vi "Test.vi"() -> ()   [LabVIEW 2015, in "PolyVIEW.lvclass"]
uses:
  PolyVIEW.lvclass
  actors/world/typedefs/markValue.ctl
  actors/world/world.lvlib
  actors/world/typedefs/markVolume.ctl
  actors/world/typedefs/markValue_cluster.ctl
  actors/world/typedefs/amountOfFood.ctl
  actors/world/typedefs/anthillType_enum.ctl
  actors/world/typedefs/worldCell_cluster.ctl
panel:
  out "Waveform Graph 3":dbl[](graph)
  out "Waveform Graph":dbl[](graph)
  out "Waveform Graph 2":dbl[][](graph)
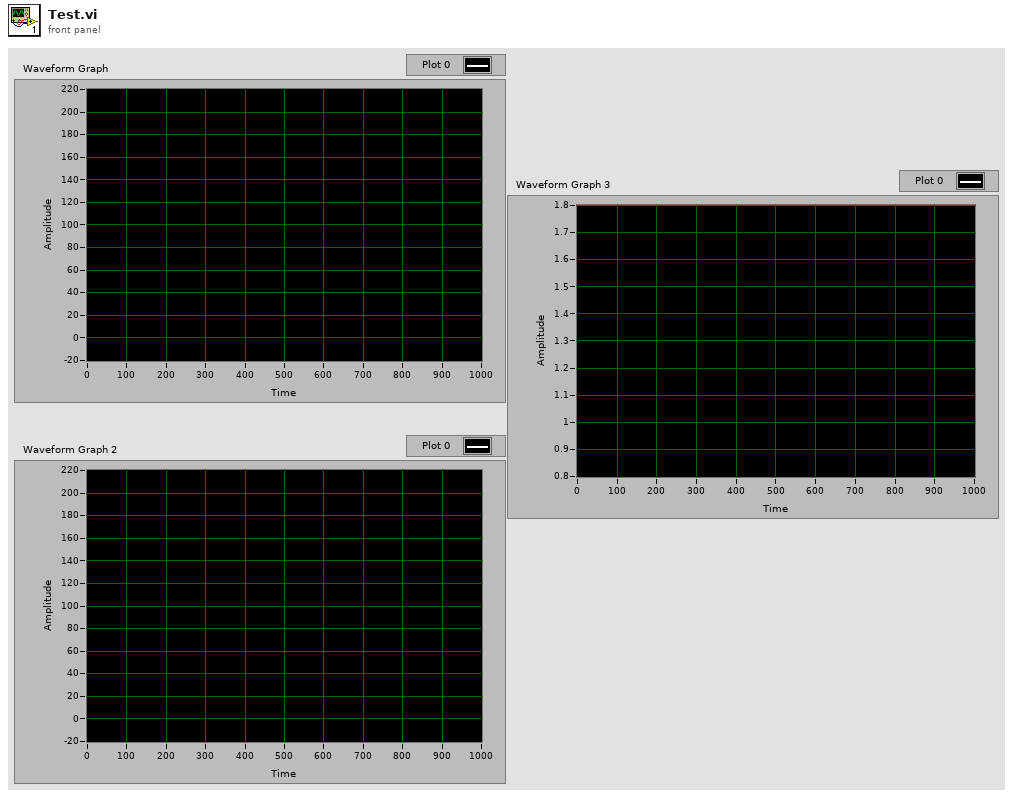
[diagram p1: front panel]
types:
  T1 = typedef "world.lvlib/worldCell_cluster.ctl" = cluster{"marksArray":T2[], "foodAmount":T5, "anthillType":T6, "absoluteHeight":u8}
  T2 = typedef "world.lvlib/markValue_cluster.ctl" = cluster{"value":T3, "volume":T4}
  T3 = typedef "world.lvlib/markValue.ctl" = u8
  T4 = typedef "world.lvlib/markVolume.ctl" = u16
  T5 = typedef "world.lvlib/amountOfFood.ctl" = i32
  T6 = typedef "world.lvlib/anthillType_enum.ctl" = enum16{"empty", "own", "rival"}
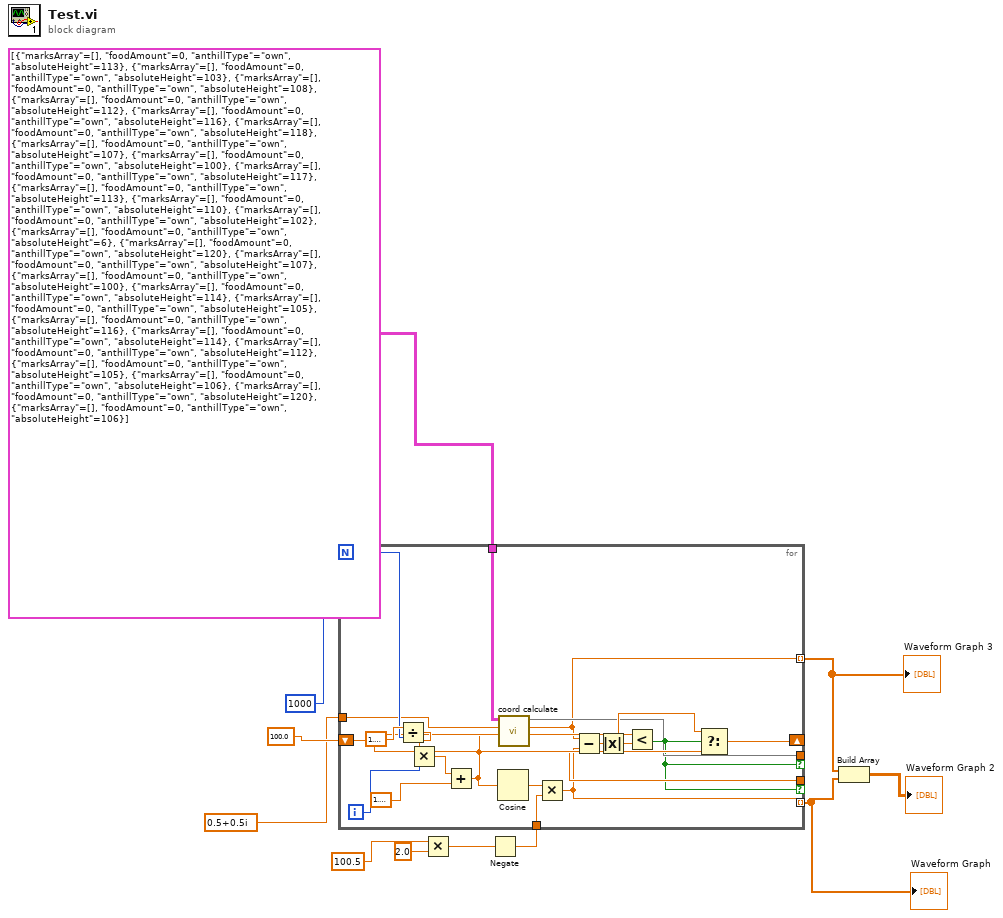
[diagram p0: block diagram]
diagram:
  n1 = Multiply(x=100.5, y=2.0) -> (x*y=w9:dbl)
  n2 = Negate(x=w9) -> (-x=w8:dbl)
  n3 = for {
    N: 1000 -> [w27]
    tunnel: w8 -> [w29]
    tunnel: T1[][] [[{"marksArray"=[], "foodAmount"=0, "anthillType"=enum."own", "absoluteHeight"=113}, {"marksArray"=[], "foodAmount"=0, "anthillType"=enum."own", "absoluteHeight"=103}, {"marksArray"=[], "foodAmount"=0, "anthillType"=enum."own", "absoluteHeight"=108}, {"marksArray"=[], "foodAmount"=0, "anthillType"=enum."own", "absoluteHeight"=112}, {"marksArray"=[], "foodAmount"=0, "anthillType"=enum."own", "absoluteHeight"=116}], [{"marksArray"=[], "foodAmount"=0, "anthillType"=enum."own", "absoluteHeight"=118}, {"marksArray"=[], "foodAmount"=0, "anthillType"=enum."own", "absoluteHeight"=107}, {"marksArray"=[], "foodAmount"=0, "anthillType"=enum."own", "absoluteHeight"=100}, {"marksArray"=[], "foodAmount"=0, "anthillType"=enum."own", "absoluteHeight"=117}, {"marksArray"=[], "foodAmount"=0, "anthillType"=enum."own", "absoluteHeight"=113}], [{"marksArray"=[], "foodAmount"=0, "anthillType"=enum."own", "absoluteHeight"=110}, {"marksArray"=[], "foodAmount"=0, "anthillType"=enum."own", "absoluteHeight"=102}, {"marksArray"=[], "foodAmount"=0, "anthillType"=enum."own", "absoluteHeight"=6}, {"marksArray"=[], "foodAmount"=0, "anthillType"=enum."own", "absoluteHeight"=120}, {"marksArray"=[], "foodAmount"=0, "anthillType"=enum."own", "absoluteHeight"=107}], [{"marksArray"=[], "foodAmount"=0, "anthillType"=enum."own", "absoluteHeight"=100}, {"marksArray"=[], "foodAmount"=0, "anthillType"=enum."own", "absoluteHeight"=114}, {"marksArray"=[], "foodAmount"=0, "anthillType"=enum."own", "absoluteHeight"=105}, {"marksArray"=[], "foodAmount"=0, "anthillType"=enum."own", "absoluteHeight"=116}, {"marksArray"=[], "foodAmount"=0, "anthillType"=enum."own", "absoluteHeight"=114}], [{"marksArray"=[], "foodAmount"=0, "anthillType"=enum."own", "absoluteHeight"=112}, {"marksArray"=[], "foodAmount"=0, "anthillType"=enum."own", "absoluteHeight"=105}, {"marksArray"=[], "foodAmount"=0, "anthillType"=enum."own", "absoluteHeight"=106}, {"marksArray"=[], "foodAmount"=0, "anthillType"=enum."own", "absoluteHeight"=120}, {"marksArray"=[], "foodAmount"=0, "anthillType"=enum."own", "absoluteHeight"=106}]] ("pieceOfWorld 3") -> [w22]
    shift-right: [w18] -> _
    shift-left: 100.0 -> [w20]
    tunnel: cdb 0.5+0.5i ("coord") -> [w17]
    tunnel: [w16] -> _ if=w14
    tunnel: [w15] -> _ if=w14
    tunnel: [w13] -> w1 mode=indexing
    tunnel: [w12] -> w3 mode=indexing
    i -> [w26]
    n4 = Divide(x=1.5707963267948966, y=w27) -> (x/y=w25:dbl)
    n5 = Multiply(x=w25, y=w26) -> (x*y=w24:dbl)
    n6 = Add(x=w24, y=1.5707963267948966) -> (x+y=w16:dbl)
    n7 = Cosine(x=w16) -> (cos(x)=w30:dbl)
    n8 = call "coord calculate.vi"("theta"=w16, "coord in"=w17, "pieceOfWorld in"=w22) -> ("coord out"=w13:cdb, 3:w15)  [unwired: 6 in, 1 out]
    n9 = Multiply(x=w30, y=w29) -> (x*y=w12:dbl)
    n10 = Subtract(x=w13, y=w12) -> (x-y=w21:cdb)
    n11 = Absolute Value(x=w21) -> (abs(x)=w19:dbl)
    n12 = Less?(x=w20, y=w19) -> (x < y?=w14:bool)
    n13 = Select(t=w19, s=w14, f=w20) -> (s? t:f=w18:dbl)
  }
  "Waveform Graph" <- w3
  "Waveform Graph 3" <- w1
  n14 = Build Array(w1, w3) -> (→"Waveform Graph 2":cdb[][])
